vi "parseRangeMode.vi"(8 "error in (no error)":errorcluster, 11 "String":string) -> (0 "error out":errorcluster, 3 "Data":dbl[](array[numeric]))   [LabVIEW 2020, in "horiba.lvlib" / "CCD.lvclass"]
doc: "Parse center wavelengths from json array into LV array."
uses:
  CCD.lvclass
  <vilib>/JDP Science/JSONtext/LVClass Serializer/JSONtext LVClass Serializer.lvclass
  CCD.lvclass/CCD.ctl
  8fe7bb78-7376-43c1-906c-2fa6ce8d17f9.vi
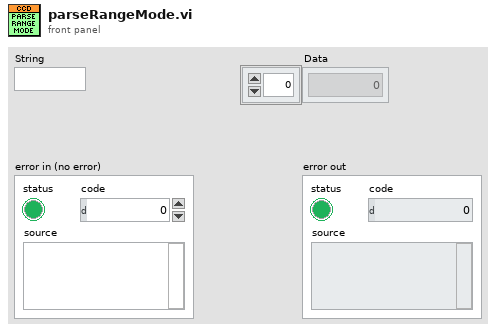
[diagram p1: front panel]
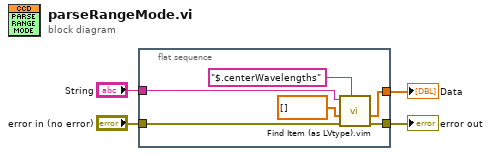
[diagram p0: block diagram]
diagram:
  n1 = flat-sequence {
    tunnel: "String" -> [w9]
    tunnel: [w7] -> w2
    tunnel: "error in (no error)" -> [w6]
    tunnel: [w5] -> w4
    frame #0 {
      n2 = call "Find Item (as LVtype).vim"("$Path or Item Name"="$.centerWavelengths", "error in (no error)"=w6, "Data Type and Default Value"=dbl[] [], "JSON"=w9) -> ("error out"=w5:errorcluster, "Data"=w7:dbl[])  [unwired: 4 in, 2 out]
    }
  }
  "error out" <- w4
  "Data" <- w2
